vi "Log Write.vi"(6 "Controller Data In":refnum<data-value>, 7 "Write Header":bool, 8 "Measurement In":refnum<data-value>, 9 "State Estimate In":refnum<data-value>, 10 "Log Handle In":T1, 11 "Error In":errorcluster) -> (0 "Measurement Out":refnum<data-value>, 1 "State Estimate Out":refnum<data-value>, 2 "Log Handle Out":T1, 3 "Error Out":errorcluster, 4 "Controller Data Out":refnum<data-value>, 5 "Logged Events":string[](array[string]))   [LabVIEW 2021]
uses:
  State Estimator/Measurements.ctl
  IMU/IMU Data.ctl
  Steering Motor Encoder/Steering Motor Encoder Data.ctl
  GNSS/GNSS Data.ctl
  State Estimator/State Estimate.ctl
  Log Handle.ctl
  Controller Data.ctl
  Drive Motor/Drive Motor Data.ctl
  Steering Motor/Steering Motor Data.ctl
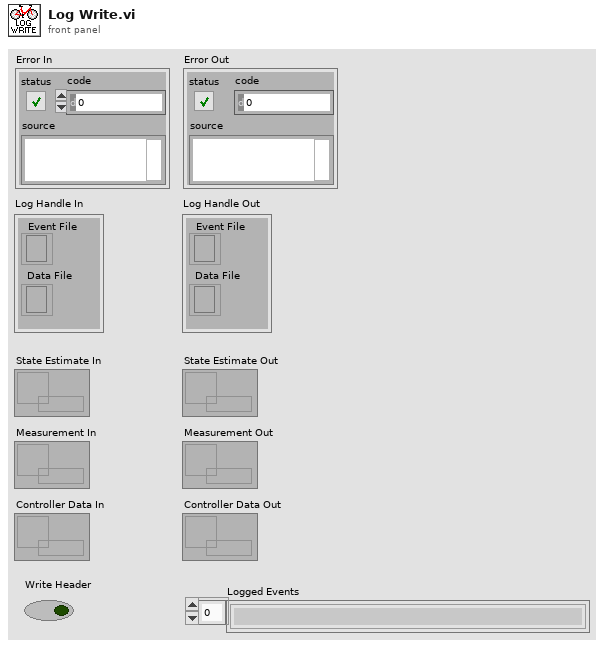
[diagram p1: front panel]
types:
  T1 = typedef "Log Handle.ctl" = cluster{"Data File":refnum<file>, "Event File":refnum<file>}
  T2 = typedef "Controller Data.ctl" = cluster{"Drive Motor Data":T3, "Steering Motor Data":T4}
  T3 = typedef "Drive Motor Data.ctl" = cluster{"Angular Speed (rad/s)":dbl, "Input Current (A)":dbl, "Motor Current (A)":dbl, "MOSFET Temperature (deg C)":dbl}
  T4 = typedef "Steering Motor Data.ctl" = cluster{"PWM":dbl, "Steering Angle Rate (rad/s)":dbl}
  T5 = typedef "State Estimate.ctl" = cluster{"X (m)":dbl, "Y (m)":dbl, "Psi (rad)":dbl, "Roll (rad)":dbl, "Roll Rate (rad/s)":dbl, "delta":dbl, "velocity":dbl}
  T6 = typedef "Measurements.ctl" = cluster{"IMU Data":T7, "Steering Motor Encoder Data":T8, "GNSS Data":T9}
  T7 = typedef "IMU Data.ctl" = cluster{"Gyroscope":cluster{"X (rad/s)":dbl, "Y (rad/s)":dbl, "Z (rad/s)":dbl}, "Accelerometer":cluster{"X (m/s^2)":dbl, "Y (m/s^2)":dbl, "Z (m/s^2)":dbl}, "Flag IMU":dbl}
  T8 = typedef "Steering Motor Encoder Data.ctl" = cluster{"Encoder Position (counts)":i32, "Steering Angle (rad)":dbl, "Flag Steering Encoder":dbl}
  T9 = typedef "GNSS Data.ctl" = cluster{"Latitude (rad)":dbl, "Longitude (rad)":dbl, "Altitude (m)":dbl, "Speed (m/s)":dbl, "Heading (rad)":dbl, "Fix Quality":i32, "Number of Satellites":i32, "Latitude (deg)":dbl, "Longitude (deg)":dbl, "Flag GNSS":dbl}
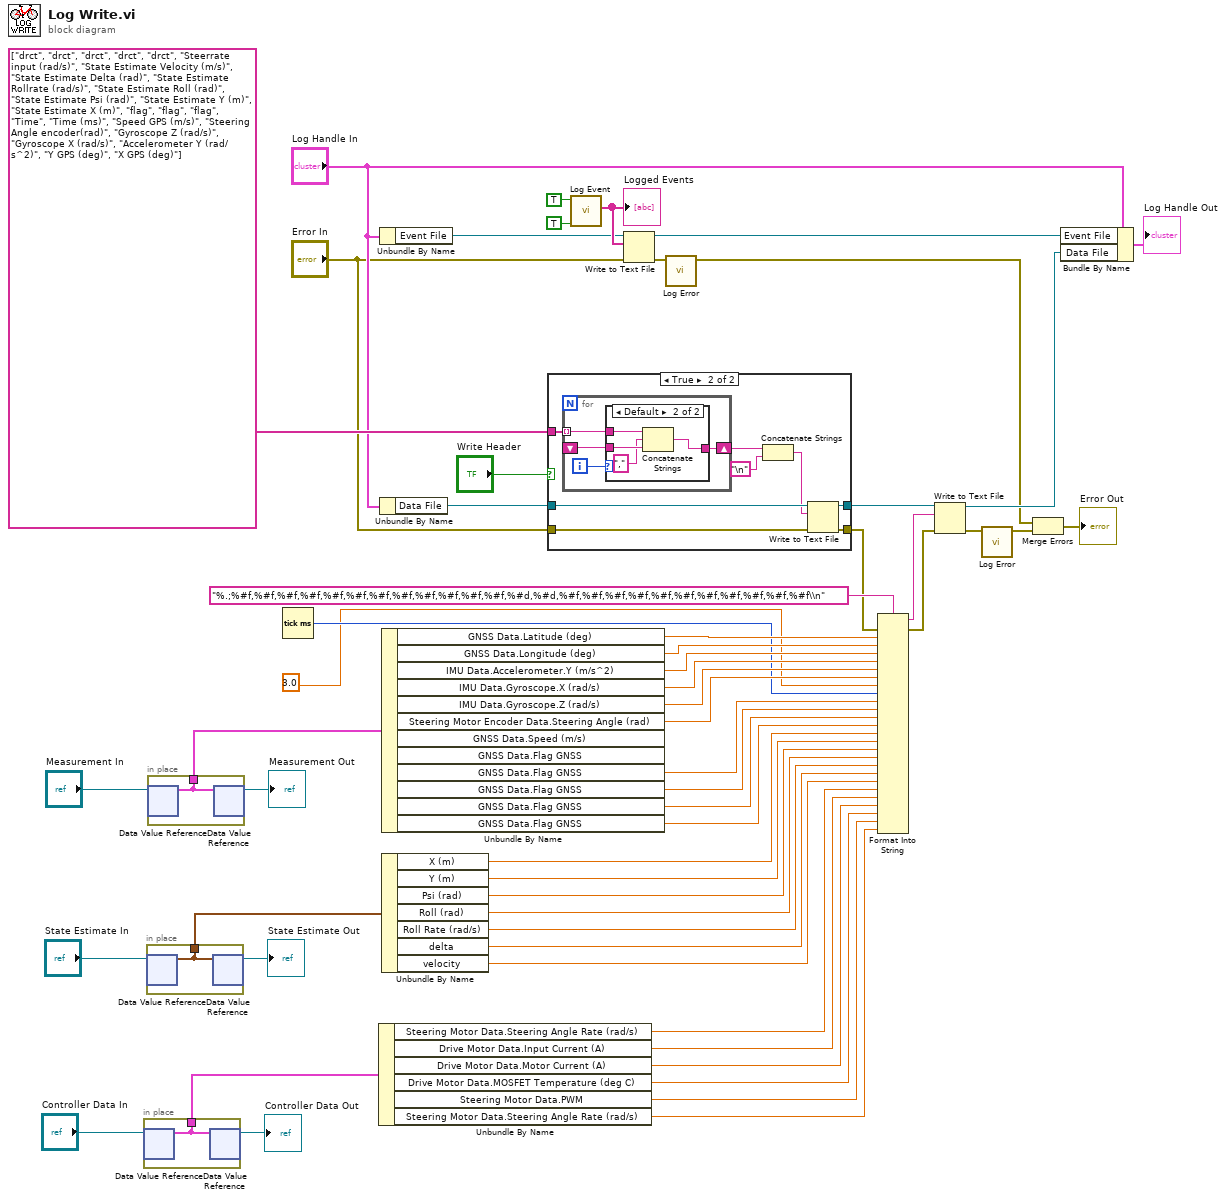
[diagram p0: block diagram]
diagram:
  n1 = in-place {
    in-place-border: [w57] -> w17
    n2 = in-place-dvr #1("Controller Data In") -> (w57:T2)  [unwired: 1 out]
    n3 = in-place-dvr #1(w57) -> (→"Controller Data Out":refnum<data-value>)  [unwired: 1 out]
  }
  n4 = in-place {
    in-place-border: [w58] -> w51
    n5 = in-place-dvr #2("State Estimate In") -> (w58:T5)  [unwired: 1 out]
    n6 = in-place-dvr #2(w58) -> (→"State Estimate Out":refnum<data-value>)  [unwired: 1 out]
  }
  n7 = in-place {
    in-place-border: [w59] -> w52
    n8 = in-place-dvr #3("Measurement In") -> (w59:T6)  [unwired: 1 out]
    n9 = in-place-dvr #3(w59) -> (→"Measurement Out":refnum<data-value>)  [unwired: 1 out]
  }
  n10 = Tick Count (ms)() -> (millisecond timer value=w10:u32)
  n11 = Unbundle By Name(w17) -> ("Steering Motor Data.Steering Angle Rate (rad/s)"=w16:dbl, "Drive Motor Data.Input Current (A)"=w15:dbl, "Drive Motor Data.Motor Current (A)"=w14:dbl, "Drive Motor Data.MOSFET Temperature (deg C)"=w13:dbl, "Steering Motor Data.PWM"=w12:dbl, "Steering Motor Data.Steering Angle Rate (rad/s)"=w11:dbl)
  n12 = Unbundle By Name("Log Handle In") -> ("Event File"=w29:refnum<file>)
  n13 = Unbundle By Name("Log Handle In") -> ("Data File"=w49:refnum<file>)
  n14 = Unbundle By Name(w52) -> ("GNSS Data.Latitude (deg)"=w47:dbl, "GNSS Data.Longitude (deg)"=w46:dbl, "IMU Data.Accelerometer.Y (m/s^2)"=w45:dbl, "IMU Data.Gyroscope.X (rad/s)"=w44:dbl, "IMU Data.Gyroscope.Z (rad/s)"=w43:dbl, "Steering Motor Encoder Data.Steering Angle (rad)"=w42:dbl, "GNSS Data.Flag GNSS"=w1:dbl, "GNSS Data.Flag GNSS"=w41:dbl, "GNSS Data.Flag GNSS"=w40:dbl, "GNSS Data.Flag GNSS"=w39:dbl)  [unwired: 2 out]
  n15 = Unbundle By Name(w51) -> ("X (m)"=w8:dbl, "Y (m)"=w7:dbl, "Psi (rad)"=w6:dbl, "Roll (rad)"=w5:dbl, "Roll Rate (rad/s)"=w4:dbl, "delta"=w3:dbl, "velocity"=w2:dbl)
  n16 = case shown="True" "Write Header" {
    tunnel: string[] ["drct", "drct", "drct", "drct", "drct", "Steerrate input (rad/s)", "State Estimate Velocity (m/s)", "State Estimate Delta (rad)", "State Estimate Rollrate (rad/s)", "State Estimate Roll (rad)", "State Estimate Psi (rad)", "State Estimate Y (m)", "State Estimate X (m)", "flag", "flag", "flag", "Time", "Time (ms)", "Speed GPS (m/s)", "Steering Angle encoder(rad)", "Gyroscope Z (rad/s)", "Gyroscope X (rad/s)", "Accelerometer Y (rad/s^2)", "Y GPS (deg)", "X GPS (deg)"] ("channel name(s) in (Untitled)") -> [_ w69]
    tunnel: w49 -> [w61 w68]
    tunnel: "Error In" -> [w60 w67]
    tunnel: [w61 w66] -> w37
    tunnel: [w60 w65] -> w35
    frame False {
    }
    frame True {
      n17 = for {
        tunnel: w69 -> [w73] mode=indexing
        shift-right: [w71] -> w64
        shift-left: _ -> [w70]
        i -> [w72]
        n18 = case shown="Default" w72 {
          tunnel: w73 -> [w74 w78]
          tunnel: [w74 w77] -> w71
          tunnel: w70 -> [_ w76]
          frame 0 {
          }
          frame Default {
            n19 = Concatenate Strings(w78, "," ("string"), w76) -> (w77:string)
          }
        }
      }
      n20 = Concatenate Strings(w64, "\n") -> (w63:string)
      n21 = Write to Text File(file (use dialog)=w68, text=w63, error in=w67) -> (refnum out=w66:refnum<file>, error out=w65:errorcluster)  [unwired: 1 in, 1 out]
    }
  }
  n22 = call "Log Event.vi"("Clear Log"=TRUE, "Read"=TRUE) -> ("All Events"=w31:string[])  [unwired: 9 in]
  "Logged Events" <- w31
  n23 = Write to Text File(file (use dialog)=w29, text=w31, error in="Error In") -> (refnum out=w26:refnum<file>, error out=w25:errorcluster)  [unwired: 1 in, 1 out]
  n24 = call "Log Error.vi"("Error In"=w25) -> ("Error Out"=w22:errorcluster)  [unwired: 10 in]
  n25 = Format Into String(format string="%.;%#f,%#f,%#f,%#f,%#f,%#f,%#f,%#f,%#f,%#f,%#f,%#f,%#d,%#d,%#f,%#f,%#f,%#f,%#f,%#f,%#f,%#f,%#f,%#f,%#f\\n", error in=w35, w47, w46, w45, w44, w43, w42, 3.0, w10, w1, w41, w40, w39, w8, w7, w6, w5, w4, w3, w2, w16, w15, w14, w13, w12, w11) -> (resulting string=w36:string, error out=w34:errorcluster)  [unwired: 1 in]
  n26 = Write to Text File(file (use dialog)=w37, text=w36, error in=w34) -> (refnum out=w27:refnum<file>, error out=w24:errorcluster)  [unwired: 1 in, 1 out]
  n27 = call "Log Error.vi"("Error In"=w24) -> ("Error Out"=w23:errorcluster)  [unwired: 10 in]
  n28 = Merge Errors(w22, w23) -> (→"Error Out":errorcluster)
  n29 = Bundle By Name(cluster="Log Handle In", "Event File"=w26, "Data File"=w27) -> (→"Log Handle Out":T1)
